vi "Dequeue.vi"(8 "error in (no error)":errorcluster, 11 "MessageQueue":refnum<queue>) -> (0 "error out":errorcluster, 1 "Message Data":variant, 2 "Message":string, 3 "MessageQueue":refnum<queue>)   [LabVIEW 2018, in "FgenModule.lvlib"]
uses:
  FgenModule.lvlib
  PublicAPI/Arguments/Messages/clMessage.ctl
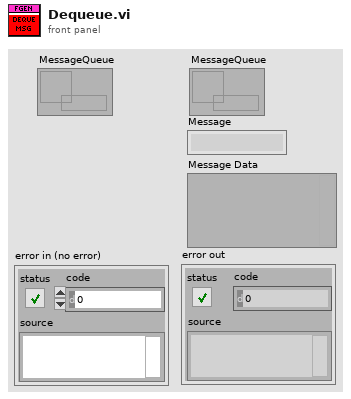
[diagram p1: front panel]
types:
  T1 = typedef "FgenModule.lvlib/clMessage.ctl" = cluster{"Message":string, "Message Data":variant}
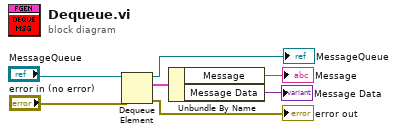
[diagram p0: block diagram]
diagram:
  n1 = Dequeue Element(queue="MessageQueue", error in (no error)="error in (no error)") -> (queue out=→"MessageQueue":refnum<queue>, element=w4:T1, error out=→"error out":errorcluster)  [unwired: 1 in, 1 out]
  n2 = Unbundle By Name(w4) -> ("Message"=→"Message":string, "Message Data"=→"Message Data":variant)
